vi "Drive Straight.vi"(2 "Max Power":dbl=0.35 format="%#_13g", 3 "output range":cluster{"output high":dbl, "output low":dbl}={"output high"=1.0, "output low"=-1.0} {"output low" format="%.2f"; "output high" format="%.2f"}, 5 "Swerve DevRef":T2[](array[typedef]), 6 "Wheel DevRef":T2[](array[typedef]), 7 "Drive Angle":dbl=3.141592653589793, 9 "Time Condition":u32=10000, 11 "Total Distance( ticks )":dbl format="%#_13g", 12 "Start Power":dbl format="%#_13g", 13 "Min Power":dbl=0.35 format="%#_13g", 14 "PID gains Rotational Correction":T1={"proportional gain (Kc)"=0.0001, "integral time (Ti, min)"=0.0, "derivative time (Td, min)"=0.0} {"derivative time (Td, min)" format="%.3f"; "integral time (Ti, min)" format="%.6f"; "proportional gain (Kc)" format="%.9f"}, 15 "error in":errorcluster) -> (4 "error out":errorcluster)   [LabVIEW 2016, in "Huskie Swerve.lvlib"]
uses:
  Huskie Swerve.lvlib
  <vilib>/Rock Robotics/WPI/MotorControl/WPI_MotorControlDeviceRef.ctl
  <vilib>/Rock Robotics/WPI/MotorControl/WPI_MotorControlType.ctl
  <vilib>/Rock Robotics/SystemInterfaces/DIO/FPGA_DIOPWMChannel.ctl
  <vilib>/Rock Robotics/WPI/PWM/WPI_PWMDeadband.ctl
  <vilib>/Analysis/baseanly.llb/Mean (DBL).vi
  <vilib>/addons/control/pid/pid.llb/PID (DBL).vi
  <vilib>/Analysis/NI_AALBase.lvlib
  <vilib>/addons/control/pid/NI_PID_pid.lvlib
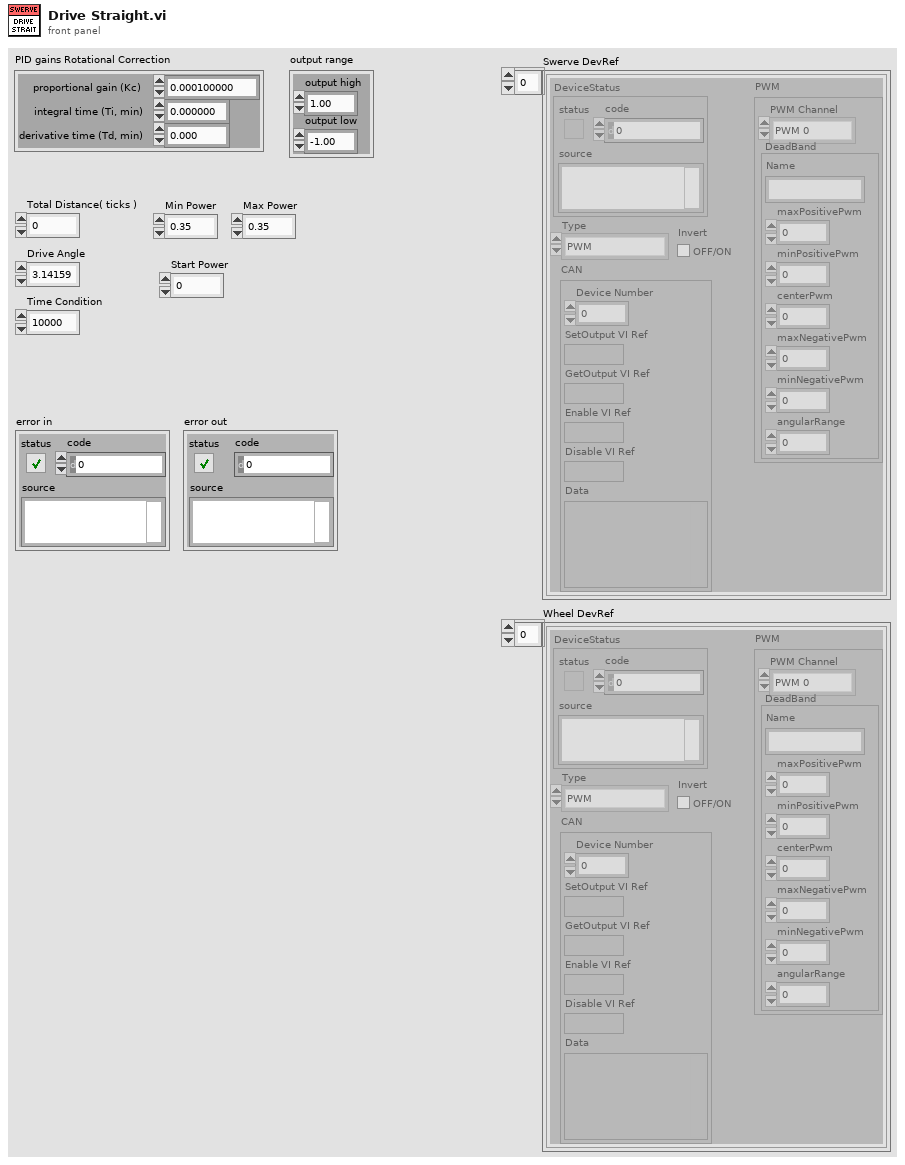
[diagram p1: front panel]
types:
  T1 = cluster{"proportional gain (Kc)":dbl, "integral time (Ti, min)":dbl, "derivative time (Td, min)":dbl}
  T2 = typedef "WPI_MotorControlDeviceRef.ctl" = cluster{"DeviceStatus":errorcluster, "Type":T3, "PWM":cluster{"PWM Channel":T4, "DeadBand":T5}, "CAN":cluster{"Device Number":u8, "SetOutput VI Ref":variant, "GetOutput VI Ref":variant, "Enable VI Ref":variant, "Disable VI Ref":variant, "Data":variant}, "Invert":bool}
  T3 = typedef "WPI_MotorControlType.ctl" = enum16{"PWM", "CAN"}
  T4 = typedef "FPGA_DIOPWMChannel.ctl" = enum8{"PWM 0", "PWM 1", "PWM 2", "PWM 3", "PWM 4", "PWM 5", "PWM 6", "PWM 7", "PWM 8", "PWM 9", "PWM MXP 0", "PWM MXP 1", "PWM MXP 2", "PWM MXP 3", "PWM MXP 4", "PWM MXP 5", "PWM MXP 6", "PWM MXP 7", "PWM MXP 8", "PWM MXP 9", "Invalid"}
  T5 = typedef "WPI_PWMDeadband.ctl" = cluster{"Name":string, "maxPositivePwm":i32, "minPositivePwm":i32, "centerPwm":i32, "maxNegativePwm":i32, "minNegativePwm":i32, "angularRange":u16}
  T6 = typedef "WPI_CANTalonSRX_GlobalStatus.ctl" = cluster{"Applied Throttle":dbl, "Module Enabled":bool, "CAN Error":errorcluster, "Closed Loop Error":dbl, "Forward Limit Switch Closed":bool, "Reverse Limit Switch Closed":bool, "Sensor Position":dbl, "Sensor Velocity":dbl, "Current":dbl, "Sticky Fault - Over Temp":bool, "Sticky Fault - Under Voltage":bool, "Sticky Fault - Forward Limit":bool, "Sticky Fault - Reverse Limit":bool, "Sticky Fault - Forward Soft Limit":bool, "Sticky Fault - Reverse Soft Limit":bool, "Brake is Enabled":bool, "Encoder Position":dbl, "Encoder Velocity":dbl, "Encoder Index Count":dbl, "Encoder A Pin State":bool, "Encoder B Pin State":bool, "Encoder Index Pin State":bool, "Analog In":dbl, "Analog In Velocity":dbl, "Temperature (C)":dbl, "Battery Voltage":dbl, "Control 5 Is Supported":bool, "Current Profile Slot Select":dbl, "Pos Div 8":bool, "Vel Div 4":bool, "Pulse Width Position":i32, "Pulse Width Velocity":i32, "Pulse Width Rise To Rise (us)":i32, "Pulse Width Rise To Fall (us)":i32, "Mot Prof Active Is Under Run":bool, "Mot Prof Active Has Under Run":bool, "Mot Prof Active Is Last":bool, "Mot Prof Active Velocity Only":bool, "Mot Prof Active Is Valid":bool, "Mot Prof Buffer Is Full":bool, "Mot Prof Active Profile Slot Select":i32, "Mot Prof NextID":i32, "Mot Prof Count":i32, "Mot Prof Active Velocity":dbl, "Mot Prof Active Position":dbl, "Mot Prof Output Enable":i32, "UsageFrame":u32, "Motion Magic Active Trajectory":cluster{"Velocity":dbl, "Position":dbl}}
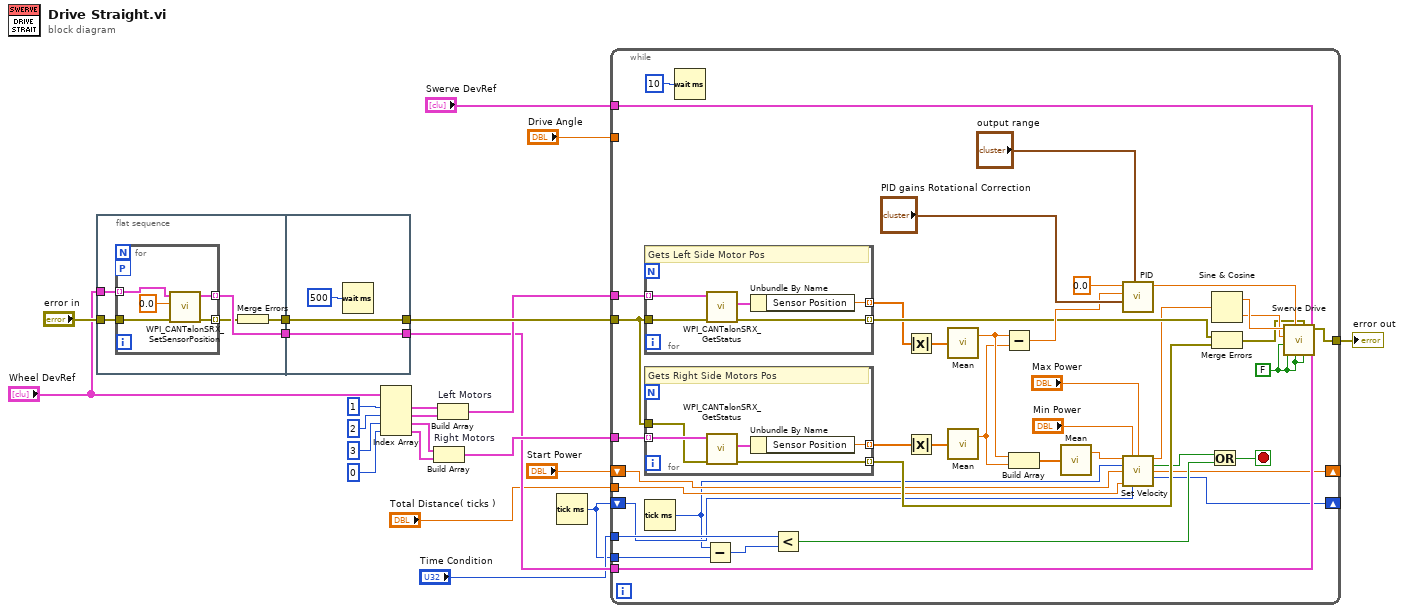
[diagram p0: block diagram]
diagram:
  n1 = flat-sequence {
    tunnel: "Wheel DevRef" -> [w28]
    tunnel: "error in" -> [w26]
    tunnel: [w27] -> w23
    tunnel: [w24] -> w22
    tunnel: [w36] -> w6
    tunnel: w23 -> [w36]
    tunnel: w22 -> [w34]
    tunnel: [w34] -> w11
    frame #0 {
      n2 = for {
        tunnel: w28 -> [w33] mode=indexing
        tunnel: [w31] -> w27 mode=indexing
        workers-P: _ -> [_]
        tunnel: w26 -> [w30]
        tunnel: [w29] -> w25 mode=indexing
        n3 = call <vilib>:"WPI_CANTalonSRX_SetSensorPosition.vi"("error in (no error)"=w30, "New Sensor Position"=0.0, "CAN Talon SRX Ref"=w33) -> ("error out"=w29:errorcluster, "CAN Talon SRX Ref"=w31:T2)  [unwired: 7 in]
      }
      n4 = Merge Errors(w25) -> (w24:errorcluster)
    }
    frame #1 {
      n5 = Wait (ms)(milliseconds to wait=u32 500) -> ()  [unwired: 1 out]
    }
  }
  n6 = Index Array(array="Wheel DevRef", index #1=1 ("index"), index #2=2 ("index"), index #3=3 ("index"), index #4=0 ("index")) -> (element #1=w15:T2, element #2=w16:T2, element #3=w13:T2, element #4=w14:T2)
  n7 = Build Array "Right Motors"(w13, w14) -> (w9:T2[])
  n8 = Build Array "Left Motors"(w15, w16) -> (w10:T2[])
  n9 = Tick Count (ms)() -> (millisecond timer value=w4:u32)
  n10 = while {
    tunnel: w11 -> [w70]
    tunnel: w10 -> [w77]
    tunnel: w9 -> [w76]
    tunnel: "Drive Angle" -> [_]
    tunnel: "Swerve DevRef" -> [w63]
    tunnel: w6 -> [w62]
    tunnel: "Time Condition" -> [w59]
    tunnel: w4 -> [w60]
    shift-right: [w55] -> _
    shift-left: "Start Power" -> [w54]
    shift-right: [w47] -> _
    shift-left: w4 -> [w44]
    tunnel: "Total Distance( ticks )" -> [w45]
    tunnel: [w38] -> w1
    stop <- w57 stop-if-true
    w37 = FALSE ("Straight Drive")
    n11 = for {
      tunnel: [w86] -> w53 mode=indexing
      tunnel: w77 -> [w85] mode=indexing
      tunnel: w70 -> [w84]
      tunnel: [w83] -> w66 mode=indexing
      # "Gets Left Side Motor Pos"
      n12 = call <vilib>:"WPI_CANTalonSRX_GetStatus.vi"("error in (no error)"=w84, "CAN Talon SRX Ref"=w85) -> ("error out"=w83:errorcluster, "Talon SRX Status"=w87:T6)  [unwired: 7 in, 1 out]
      n13 = Unbundle By Name(w87) -> ("Sensor Position"=w86:dbl)
    }
    n14 = for {
      tunnel: [w81] -> w52 mode=indexing
      tunnel: w76 -> [w80] mode=indexing
      tunnel: w70 -> [w79]
      tunnel: [w78] -> w65 mode=indexing
      # "Gets Right Side Motors Pos"
      n15 = call <vilib>:"WPI_CANTalonSRX_GetStatus.vi"("error in (no error)"=w79, "CAN Talon SRX Ref"=w80) -> ("error out"=w78:errorcluster, "Talon SRX Status"=w82:T6)  [unwired: 7 in, 1 out]
      n16 = Unbundle By Name(w82) -> ("Sensor Position"=w81:dbl)
    }
    n17 = Tick Count (ms)() -> (millisecond timer value=w43:u32)
    n18 = Wait (ms)(milliseconds to wait=u32 10) -> ()  [unwired: 1 out]
    n19 = Subtract(x=w43, y=w60) -> (x-y=w61:u32)
    n20 = Less?(x=w59, y=w61) -> (x < y?=w58:bool)
    n21 = Absolute Value(x=w53) -> (abs(x)=w42:dbl[])
    n22 = Absolute Value(x=w52) -> (abs(x)=w41:dbl[])
    n23 = call-poly <vilib>:"Mean.vi"("X"=w42) -> ("mean"=w51:dbl)  [unwired: 1 out]
    n24 = call-poly <vilib>:"Mean.vi"("X"=w41) -> ("mean"=w50:dbl)  [unwired: 1 out]
    n25 = Subtract(x=w51, y=w50) -> (x-y=w71:dbl)
    n26 = Build Array(w51, w50) -> (w49:dbl[])
    n27 = call-poly <vilib>:"Mean.vi"("X"=w49) -> ("mean"=w48:dbl)  [unwired: 1 out]
    n28 = call-poly <vilib>:"PID.vi"("output range"="output range", "PID gains"="PID gains Rotational Correction", "process variable"=w71, "setpoint"=0.0) -> ("output"=w67:dbl)  [unwired: 6 in, 1 out]
    n29 = call "Set Velocity.vi"("Process Variable(x)"=w48, "Min Power"="Min Power", "Max Power"="Max Power", "Current TIme"=w43, "Current Power"=w54, "Total Distance"=w45, "Last Time Input"=w44) -> ("Coerced Motor power"=w46:dbl, "End Loop?"=w56:bool, "Non-Coerced Motor Power"=w55:dbl, "Last Time Output"=w47:u32)  [unwired: 5 in]
    n30 = Or(x=w56, y=w58) -> (x .or. y?=w57:bool)
    n31 = Sine & Cosine(0:w46) -> (1:w69:dbl, 2:w68:dbl)
    n32 = Merge Errors(w66, w65) -> (w64:errorcluster)
    n33 = call "Swerve Drive.vi"("Drive Dev Ref"=w62, "Swerve Dev Ref"=w63, "X Drive"=w37, "error in"=w64, "Low Sensitivity"=w37, "Z"=w67, "Reverse Drive"=w37, "Straight Drive"=w37, "Y"=w68, "X"=w69) -> ("error out"=w38:errorcluster)  [unwired: 1 in]
  }
  "error out" <- w1
